vi "Read Line Rate - With One Method - Returns Total Value.vi"() -> ()   [LabVIEW 2017, in "Cobertura.Tests.lvlib" / "Class.lvlib"]
uses:
  Class.lvlib
  Cobertura/Class/Class.lvclass/Class.ctl
  Cobertura/Class/Read Line Rate.vi
  <vilib>/PNR/Transparent Assertions/Transparent Assertions/Transparent Assertions.lvlib
  Cobertura/Class/Class.lvclass
  Cobertura/Method/Method.lvclass
panel:
  out "error out":errorcluster
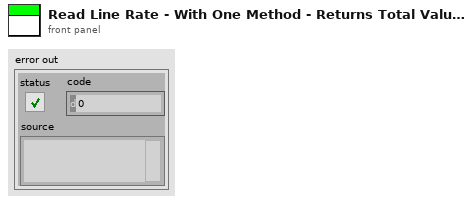
[diagram p1: front panel]
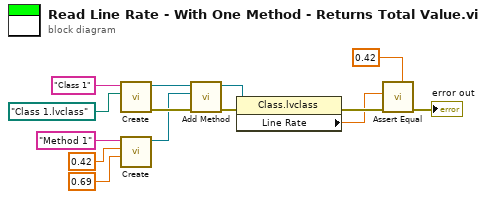
[diagram p0: block diagram]
diagram:
  n1 = call "Create.vi"("Filename"=path "Class 1.lvclass", "Name"="Class 1") -> ("error out"=w13:errorcluster, "Class"=w7:refnum<class "Class.lvclass">)  [unwired: 8 in]
  n2 = call "Create.vi"("Branch Rate"=0.69, "Line Rate"=0.42, "Name"="Method 1") -> ("Method"=w2:refnum<class "Method.lvclass">)  [unwired: 7 in, 1 out]
  n3 = call "Add Method.vi"("error in (no error)"=w13, "Method"=w2, "Class in"=w7) -> ("error out"=w8:errorcluster, "Class out"=w6:refnum<class "Class.lvclass">)  [unwired: 7 in]
  n4 = property class="Class.lvclass"(reference=w6, error in=w8) -> (error out=w12:errorcluster, "Line Rate"=w11:dbl)  [unwired: 1 out]
  n5 = call <vilib>:"Assert Equal.vi"("Expected"=0.42 ("Line Rate"), "error in (no error)"=w12, "Actual"=w11) -> ("error out"=→"error out":errorcluster)  [unwired: 8 in]
